vi "niFPGA LM Resampler.vi"(8 "FIFOIsFull":bool, 9 "datain":fxp<+/-,16,1>, 10 "dataRDYIn":bool, 11 "reset":bool) -> (1 "idle":bool, 2 "dataRDYOut":bool, 3 "y":fxp<+/-,18,1> format="%.18g")   [LabVIEW 2017]
uses:
  <vilib>/rvi/Emulation/niFpgaSctlEmulationGetInTimedLoop.vi
  <vilib>/Utility/error.llb/Clear Errors.vi
  <vilib>/rvi/Emulation/niFpgaSctlEmulationResourceMgr.vi
  <vilib>/rvi/Memory/Memory_Emulation/nirvimemoryEmulationManagerCache_SetValue.vi
  <vilib>/rvi/Emulation/niFpgaEmulationIsFPGAContextNoSignature.vi
  <vilib>/rvi/Memory/Memory_Emulation/nirvimemoryEmulationManagerCache_GetValue.vi
  <vilib>/rvi/Memory/Memory_Emulation/nirvimemoryEmulationManagerCache_ReleaseExclusive.vi
  <vilib>/rvi/Memory/Memory_Emulation/nirvimemoryEmulationManagerCache_InsertValue.vi
  <vilib>/rvi/Memory/Memory_Emulation/niFpgaMemoryEmulationValidateCache.vi
  <vilib>/rvi/Memory/Memory_Emulation/nirvimemoryEmulationManagerCache_MakeExclusive.vi
  <vilib>/rvi/Memory/Memory_Emulation/niFpgaMemoryEmulationCacheClearOnFirstRun.vi
  <vilib>/rvi/DataTransferAndStorage/Container/Common/niFpgaContainerGetUniqueNameForEmu.vi
  <vilib>/rvi/Emulation/niFpgaProcessEmulError.vi
  <vilib>/rvi/errors/nirviReportUnexpectedCaseInternalError (U32).vi
  <vilib>/rvi/DataTransferAndStorage/Container/Common/niFpgaContainerExecOnDevCompGetState.vi
  <vilib>/rvi/eio/common/nirviEmuReportErrorAndStop.vi
  <vilib>/rvi/DataTransferAndStorage/Container/Common/niFpgaContainerSetEmuInfo.vi
  <vilib>/rvi/DataTransferAndStorage/Container/XNode/niFpgaContainer.xnode
  <vilib>/rvi/Memory/Memory_Emulation/niFpgaMemoryEmulationRefIn.vi
  <vilib>/rvi/FXPMathLib/FxpMul/XNode/nifxpmath_Multiplier.xnode
  <vilib>/rvi/LocalResourceManager/LocalResourceManager.xnode
  <vilib>/rvi/FXPMathLib/sim/FxpSim.dll
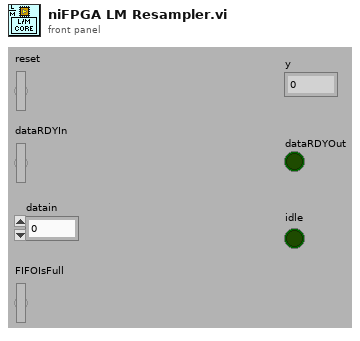
[diagram p1: front panel]
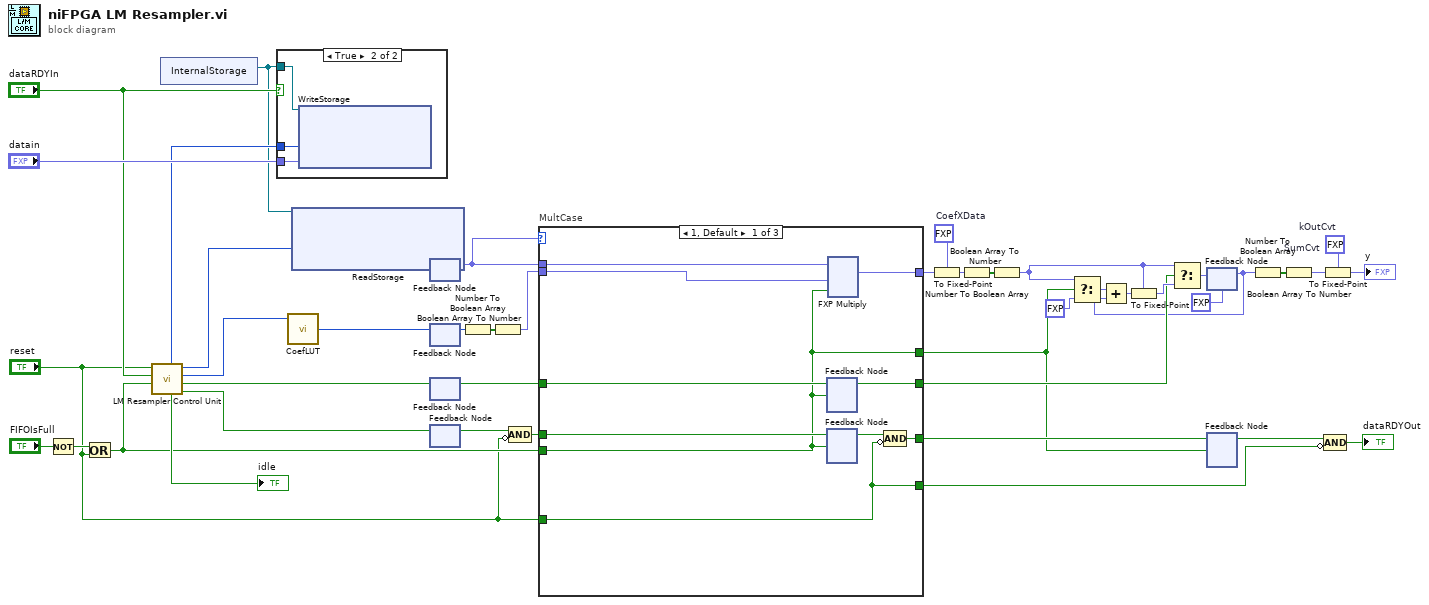
[diagram p0: block diagram]
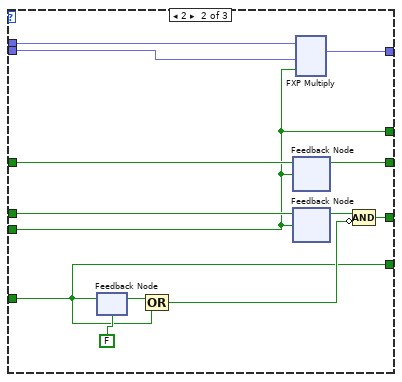
[diagram p2: hidden frame]
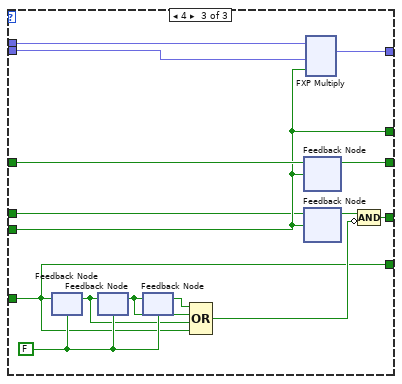
[diagram p3: hidden frame]
diagram:
  w29 = fxp<+/-,18,1> 0.0  # kOutCvt
  w34 = fxp<+/-,32,10> 0.0  # CoefXData
  n1 = Not(x="FIFOIsFull") -> (.not. x?=w42:bool)
  n2 = Or(x=w42, y="reset") -> (x .or. y?=w32:bool)
  n3 = call "LM Resampler Control Unit"("enable"=w32, "dataRDYIn"="dataRDYIn", "reset"="reset") -> ("dataReady?"=w21:bool, "clear acc?"=w19:bool, "coefIdx"=w25:u16, "dataIdx"=w33:u16, "idle?"=→"idle":bool, "memWRAddr"=w31:u16)  [unwired: 3 in]
  n4 = xnode "InternalStorage"() -> ("Memory Out"=w1:refnum<k21>)
  n5 = case "TopCASE" shown="True" "dataRDYIn" {
    tunnel: w31 -> [_ w47]
    tunnel: "datain" -> [_ w46]
    tunnel: w1 -> [_ w45]
    frame False {
    }
    frame True {
      n6 = xnode "WriteStorage"("Address"=w47, "Data"=w46, "Memory In"=w45) -> ()  [unwired: 1 out]
    }
  }
  n7 = call "CoefLUT"("address"=w25) -> ("data out"=w17:i16)  [unwired: 8 in]
  n8 = xnode "ReadStorage"("Address"=w33, "Memory In"=w1) -> ("Data"=w36:fxp<+/-,16,1>)  [unwired: 1 out]
  n9 = feedback-in #1(w36) -> ()
  n10 = feedback #1() -> (w28:fxp<+/-,16,1>)  [unwired: 1 out]
  n11 = feedback-in #2(w17) -> ()
  n12 = feedback #2() -> (w16:i16)  [unwired: 1 in]
  n13 = feedback #3() -> (w18:bool)  [unwired: 1 in]
  n14 = feedback-in #3(w19) -> ()
  n15 = feedback #4() -> (w20:bool)  [unwired: 1 in]
  n16 = feedback-in #4(w21) -> ()
  n17 = Number To Boolean Array(number=w16) -> (Boolean array=w24:bool[])
  n18 = Boolean Array To Number ("CoefCvt")(Boolean array=w24) -> (number=w23:fxp<+/-,16,1>)
  n19 = Compound Arithmetic op=AND(w20, invert "reset") -> (w27:bool)
  n20 = case "MultCase" shown="1, Default" w28 {
    tunnel: w28 -> [w57 w70 w85]
    tunnel: w23 -> [w56 w69 w84]
    tunnel: [w55 w68 w83] -> w38
    tunnel: [w48 w58 w74] -> w6
    tunnel: [w54 w67 w82] -> w15
    tunnel: "reset" -> [w53 w63 w76]
    tunnel: w32 -> [w50 w60 w73]
    tunnel: [w50 w60 w73] -> w2
    tunnel: w18 -> [w51 w62 w75]
    tunnel: w27 -> [w52 w61 w72]
    tunnel: [w53 w63 w76] -> w26
    frame 1, Default {
      n21 = feedback #5() -> (w48:bool)  [unwired: 1 in]
      n22 = feedback-in #5(w51, w50) -> ()
      n23 = feedback #6() -> (w49:bool)  [unwired: 1 in]
      n24 = feedback-in #6(w52, w50) -> ()
      n25 = xnode ("FXP Multiply")("x"=w57, "y"=w56, "input valid"=w50) -> ("x*y"=w55:fxp<+/-,32,2>)  [unwired: 1 in, 2 out]
      n26 = Compound Arithmetic op=AND(w49, invert w53) -> (w54:bool)
    }
    frame 2 {
      n27 = feedback-in #7(w63) -> ()
      n28 = feedback #7(FALSE) -> (w66:bool)
      n29 = Compound Arithmetic op=OR(w66, w63) -> (w64:bool)
      n30 = feedback #8() -> (w58:bool)  [unwired: 1 in]
      n31 = feedback-in #8(w62, w60) -> ()
      n32 = feedback #9() -> (w59:bool)  [unwired: 1 in]
      n33 = feedback-in #9(w61, w60) -> ()
      n34 = xnode ("FXP Multiply")("x"=w70, "y"=w69, "input valid"=w60) -> ("x*y"=w68:fxp<+/-,32,2>)  [unwired: 1 in, 2 out]
      n35 = Compound Arithmetic op=AND(w59, invert w64) -> (w67:bool)
    }
    frame 4 {
      w81 = FALSE
      n36 = feedback-in #10(w76) -> ()
      n37 = feedback #10(w81) -> (w80:bool)
      n38 = feedback-in #11(w80) -> ()
      n39 = feedback #11(w81) -> (w79:bool)
      n40 = feedback-in #12(w79) -> ()
      n41 = feedback #12(w81) -> (w78:bool)
      n42 = Compound Arithmetic op=OR(w78, w79, w80, w76) -> (w77:bool)
      n43 = feedback #13() -> (w74:bool)  [unwired: 1 in]
      n44 = feedback-in #13(w75, w73) -> ()
      n45 = feedback #14() -> (w71:bool)  [unwired: 1 in]
      n46 = feedback-in #14(w72, w73) -> ()
      n47 = xnode ("FXP Multiply")("x"=w85, "y"=w84, "input valid"=w73) -> ("x*y"=w83:fxp<+/-,32,2>)  [unwired: 1 in, 2 out]
      n48 = Compound Arithmetic op=AND(w71, invert w77) -> (w82:bool)
    }
  }
  n49 = To Fixed-Point(fixed-point type=w34, number=w38) -> (fixed-point=w39:fxp<+/-,32,10>)
  n50 = Number To Boolean Array(number=w39) -> (Boolean array=w40:bool[])
  n51 = Boolean Array To Number(Boolean array=w40) -> (number=w7:fxp<+/-,32,32>)
  n52 = Select(t=w7, s=w2, f=fxp<+/-,32,32> 0.0) -> (s? t:f=w8:fxp<+/-,32,32>)
  n53 = feedback #15(fxp<+/-,32,32> 0.0 ("f")) -> (w3:fxp<+/-,32,32>)
  n54 = Add(x=w8, y=w3) -> (x+y=w13:fxp<+/-,33,33>)
  n55 = To Fixed-Point(fixed-point type=w7, number=w13) -> (fixed-point=w11:fxp<+/-,32,32>)
  n56 = Select(t=w7, s=w6, f=w11) -> (s? t:f=w9:fxp<+/-,32,32>)
  n57 = feedback-in #15(w9) -> ()
  n58 = feedback #16() -> (w14:bool)  [unwired: 1 in]
  n59 = feedback-in #16(w15, w2) -> ()
  n60 = Number To Boolean Array(number=w3) -> (Boolean array=w30:bool[])
  n61 = Boolean Array To Number "SumCvt"(Boolean array=w30) -> (number=w4:fxp<+/-,32,17>)
  n62 = To Fixed-Point(fixed-point type=w29, number=w4) -> (fixed-point=→"y":fxp<+/-,18,1>)
  n63 = Compound Arithmetic op=AND(w14, invert w26) -> (→"dataRDYOut":bool)
